vi "Write Configuration File.vi"(8 "error in (no error)":errorcluster, 11 "Inst.Krohn-Hite-7008 in":refnum<class "Inst.Krohn-Hite-7008.lvclass">) -> (0 "error out":errorcluster, 3 "Inst.Krohn-Hite-7008 out":refnum<class "Inst.Krohn-Hite-7008.lvclass">)   [LabVIEW 2019, in "Inst.Krohn-Hite-7008.lvclass"]
uses:
  Inst.Krohn-Hite-7008.lvclass
  <userlib>/LevyLab/Instrument Framework/Instrument Types/VSource/Instrument.VSource.lvclass
  <userlib>/LevyLab/Configuration/Configuration.lvclass
  <userlib>/LevyLab/Instrument Framework/Instrument/Instrument.lvclass
  C:/Program Files (x86)/National Instruments/LabVIEW 2019/user.lib/LevyLab/Instrument Framework/Instrument/Instrument.lvclass
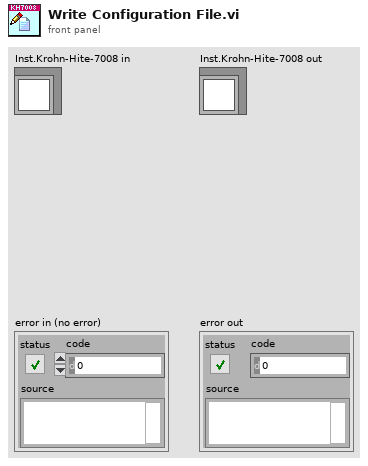
[diagram p1: front panel]
types:
  T1 = typedef "Inst.Krohn-Hite-7008.lvclass/Inst.Krohn-Hite-7008.device--Cluster.ctl" = cluster{"model":string, "device_id":string}
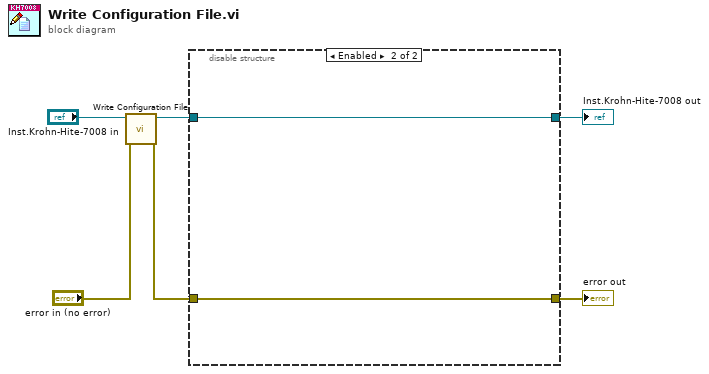
[diagram p0: block diagram]
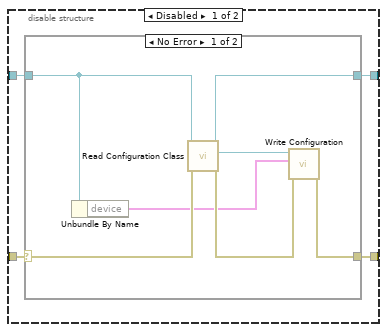
[diagram p2: hidden frame]
diagram:
  n1 = call-parent "Write Configuration File.vi"("error in (no error)"="error in (no error)", "Instrument in"="Inst.Krohn-Hite-7008 in") -> ("error out"=w4:errorcluster, "Instrument out"=w2:refnum<class "Inst.Krohn-Hite-7008.lvclass">)  [unwired: 8 in]
  n2 = disable-structure shown="Enabled" {
    disable-tunnel: [w9 w20] -> w6
    disable-tunnel: w4 -> [w8 w20]
    disable-tunnel: w2 -> [w7 w21]
    disable-tunnel: [w10 w21] -> w1
    frame Disabled {
      n3 = case shown="No Error" w8 {
        selector: w8 -> [w13 w19]
        tunnel: w7 -> [w12 w18]
        tunnel: [w16 w18] -> w10
        tunnel: [w15 w19] -> w9
        frame No Error {
          n4 = Unbundle By Name(w12) -> ("device"=w11:T1)
          n5 = call <userlib>:"Read Configuration Class.vi"("error in (no error)"=w13, "Instrument in"=w12) -> ("error out"=w17:errorcluster, "Configuration"=w14:refnum<class "Configuration.lvclass">, "Instrument out"=w16:refnum<class "Inst.Krohn-Hite-7008.lvclass">)  [unwired: 7 in]
          n6 = call <userlib>:"Write Configuration.vi"("error in (no error)"=w17, "Variant"=w11, "Configuration in"=w14) -> ("error out"=w15:errorcluster)  [unwired: 7 in, 1 out]
        }
        frame Error {
        }
      }
    }
    frame Enabled {
    }
  }
  "Inst.Krohn-Hite-7008 out" <- w1
  "error out" <- w6
